vi "HB_SetTime.vi"(8 "error in (no error)":errorcluster, 10 "Time Stamp":timestamp, 11 "HBDeviceRef":T1) -> (0 "error IO":errorcluster, 3 "HBDeviceRef":T1)   [LabVIEW 2016]
doc: "Sets the time on the Huskie Board to the specified time. This VI is automatically invoked by the HB_OpenFile VI and the current time of the roboRIO is specified. In order for the roboRIO to have the proper tine, it must be connected to the Dashboard."
uses:
  <vilib>/Rock Robotics/WPI/SerialPort/WPI_SerialPortRef.ctl
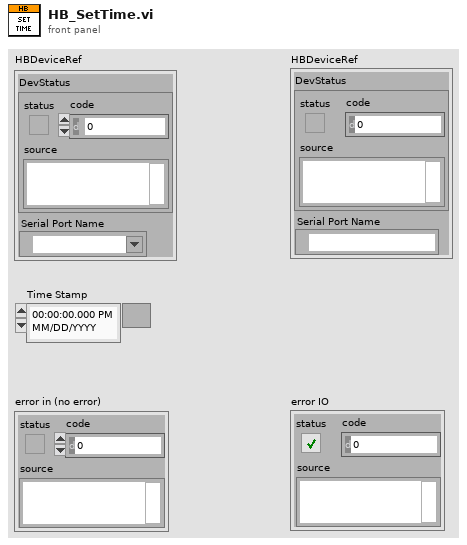
[diagram p1: front panel]
types:
  T1 = typedef "WPI_SerialPortRef.ctl" = cluster{"DevStatus":errorcluster, "Serial Port Name":refnum<visa-resource-name>}
  T2 = typedef "LVDateTimeRec.ctl" = cluster{"fractional second":dbl, "second":i32, "minute":i32, "hour":i32, "day of month":i32, "month":i32, "year":i32, "day of week":i32, "day of year":i32, "DST":i32}
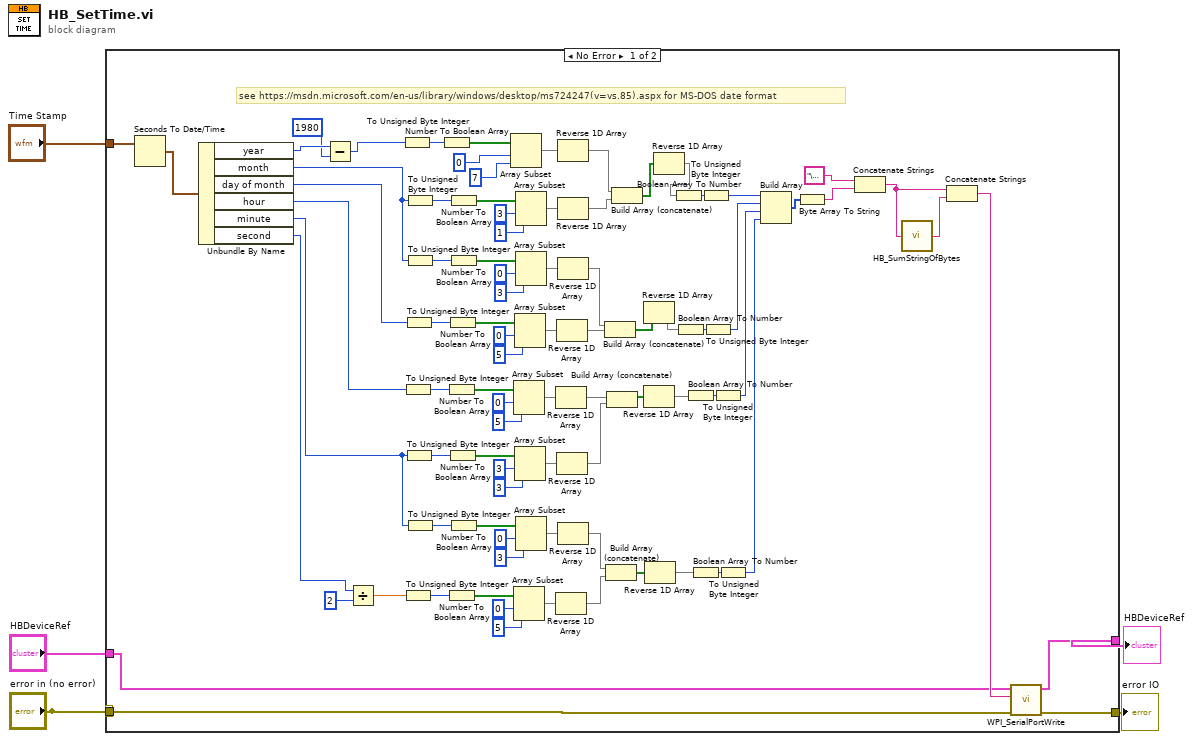
[diagram p0: block diagram]
diagram:
  n1 = case shown="No Error" "error in (no error)" {
    selector: "error in (no error)" -> [w19 w92]
    tunnel: "HBDeviceRef" -> [w16 w93]
    tunnel: "error in (no error)" -> [_ _]
    tunnel: [w17 w93] -> w2
    tunnel: [w18 w92] -> w3
    tunnel: "Time Stamp" -> [w73 _]
    frame No Error {
      # "see https://msdn.microsoft.com/en-us/library/windows/desktop/ms724247(v=vs.85).aspx for MS-DOS date format"
      n2 = Seconds To Date/Time(time stamp (now)=w73) -> (date time rec=w72:T2)  [unwired: 1 in]
      n3 = Unbundle By Name(w72) -> ("year"=w71:i32, "month"=w22:i32, "day of month"=w48:i32, "hour"=w47:i32, "minute"=w23:i32, "second"=w46:i32)
      n4 = Subtract(x=w71, y=1980) -> (x-y=w69:i32)
      n5 = Divide(x=w46, y=2) -> (x/y=w45:dbl)
      n6 = To Unsigned Byte Integer(number=w69) -> (unsigned 8bit integer=w82:u8)
      n7 = To Unsigned Byte Integer(number=w47) -> (unsigned 8bit integer=w63:u8)
      n8 = To Unsigned Byte Integer(number=w45) -> (unsigned 8bit integer=w53:u8)
      n9 = To Unsigned Byte Integer(number=w48) -> (unsigned 8bit integer=w68:u8)
      n10 = To Unsigned Byte Integer(number=w23) -> (unsigned 8bit integer=w58:u8)
      n11 = To Unsigned Byte Integer(number=w22) -> (unsigned 8bit integer=w87:u8)
      n12 = To Unsigned Byte Integer(number=w22) -> (unsigned 8bit integer=w40:u8)
      n13 = To Unsigned Byte Integer(number=w23) -> (unsigned 8bit integer=w31:u8)
      n14 = Number To Boolean Array(number=w82) -> (Boolean array=w81:bool[])
      n15 = Number To Boolean Array(number=w63) -> (Boolean array=w59:bool[])
      n16 = Number To Boolean Array(number=w53) -> (Boolean array=w49:bool[])
      n17 = Number To Boolean Array(number=w68) -> (Boolean array=w64:bool[])
      n18 = Number To Boolean Array(number=w58) -> (Boolean array=w54:bool[])
      n19 = Number To Boolean Array(number=w87) -> (Boolean array=w83:bool[])
      n20 = Number To Boolean Array(number=w40) -> (Boolean array=w36:bool[])
      n21 = Number To Boolean Array(number=w31) -> (Boolean array=w27:bool[])
      n22 = Array Subset(array=w81, index=0, length=7) -> (w14:bool[])
      n23 = Array Subset(array=w59, index=0, length=5) -> (w60:bool[])
      n24 = Array Subset(array=w49, index=0, length=5) -> (w50:bool[])
      n25 = Array Subset(array=w64, index=0, length=5) -> (w65:bool[])
      n26 = Array Subset(array=w54, index=3, length=3) -> (w55:bool[])
      n27 = Array Subset(array=w83, index=3, length=1) -> (w84:bool[])
      n28 = Array Subset(array=w36, index=0, length=3) -> (w37:bool[])
      n29 = Array Subset(array=w27, index=0, length=3) -> (w28:bool[])
      n30 = Reverse 1D Array(array=w60) -> (reversed array=w32:bool[])
      n31 = Reverse 1D Array(array=w50) -> (reversed array=w24:bool[])
      n32 = Reverse 1D Array(array=w65) -> (reversed array=w34:bool[])
      n33 = Reverse 1D Array(array=w55) -> (reversed array=w26:bool[])
      n34 = Reverse 1D Array(array=w14) -> (reversed array=w15:bool[])
      n35 = Reverse 1D Array(array=w84) -> (reversed array=w76:bool[])
      n36 = Reverse 1D Array(array=w37) -> (reversed array=w35:bool[])
      n37 = Reverse 1D Array(array=w28) -> (reversed array=w25:bool[])
      n38 = Build Array (concatenate)(w35, w34) -> (w11:bool[])
      n39 = Build Array (concatenate)(w25, w24) -> (w7:bool[])
      n40 = Build Array (concatenate)(w32, w26) -> (w9:bool[])
      n41 = Build Array (concatenate)(w15, w76) -> (w13:bool[])
      n42 = Reverse 1D Array(array=w11) -> (reversed array=w10:bool[])
      n43 = Reverse 1D Array(array=w9) -> (reversed array=w8:bool[])
      n44 = Reverse 1D Array(array=w7) -> (reversed array=w6:bool[])
      n45 = Reverse 1D Array(array=w13) -> (reversed array=w12:bool[])
      n46 = Boolean Array To Number(Boolean array=w12) -> (number=w79:u32)
      n47 = Boolean Array To Number(Boolean array=w10) -> (number=w43:u32)
      n48 = Boolean Array To Number(Boolean array=w8) -> (number=w42:u32)
      n49 = Boolean Array To Number(Boolean array=w6) -> (number=w41:u32)
      n50 = To Unsigned Byte Integer(number=w79) -> (unsigned 8bit integer=w78:u8)
      n51 = To Unsigned Byte Integer(number=w43) -> (unsigned 8bit integer=w33:u8)
      n52 = To Unsigned Byte Integer(number=w42) -> (unsigned 8bit integer=w21:u8)
      n53 = To Unsigned Byte Integer(number=w41) -> (unsigned 8bit integer=w20:u8)
      n54 = Build Array(w78, w33, w21, w20) -> (w77:u8[])
      n55 = Byte Array To String(unsigned byte array=w77) -> (string=w75:string)
      n56 = Concatenate Strings("\u0005", w75) -> (w89:string)
      n57 = call <vilib>:"HB_SumStringOfBytes.vi"("String Of Bytes"=w89) -> ("Sum as String"=w88:string)
      n58 = Concatenate Strings(w89, w88) -> (w90:string)
      n59 = call <vilib>:"WPI_SerialPortWrite.vi"("error in (no error)"=w19, "Buffer"=w90, "SerialPortRef"=w16) -> ("error out"=w18:errorcluster, "SerialPortRef"=w17:T1)  [unwired: 6 in, 1 out]
    }
    frame Error {
    }
  }
  "HBDeviceRef" <- w2
  "error IO" <- w3
